vi "HEWH Update Station Message Heating.vi"(6 "Test Complete":bool, 8 "error in (no error)":errorcluster, 10 "Station Label":string, 11 "Display Data (RLT)":T1 {"Current Display" format="%.2f"; "Cycle Count Display" format="%04d"}) -> (0 "error out":errorcluster)   [LabVIEW 2016]
uses:
  Utility/Save File/Public/Type Definitions/Save File Appliance Display.ctl
  Utility/Save File/Public/Type Definitions/Save File Unit Type.ctl
  Utility/Type Definitions/UTILITY Notifier.ctl
  Utility/Custom Pallet Controls/Custom Pallet String.ctl
  Utility/Save File/Global/Save File Globals HCC.vi
  Utility/Save File/Save File.lvlib
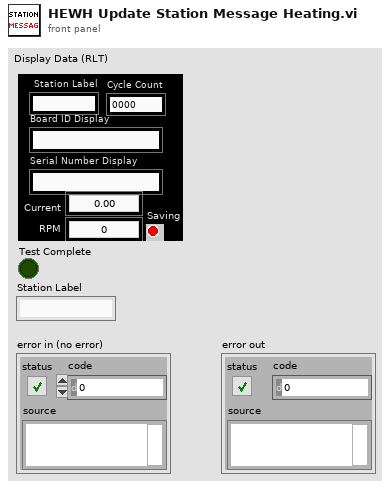
[diagram p1: front panel]
types:
  T1 = typedef "Save File Appliance Display.ctl" = cluster{"Status Color":u32, "Serial Number Display":string, "Cycle Count Display":i32, "Station Label Display":string, "Current Run Start Time Display":dbl, "Board ID Display":string, "RPM Display":u32, "Current Display":dbl, "Current Path Display":path, "Saving Display":bool, "Unit Type Display":T2, "Total Time On Display":dbl, "UI Button":bool}
  T2 = typedef "Save File.lvlib/Save File Unit Type.ctl" = enum32{"", "Viper", "Hawk", "2015"}
  T3 = typedef "UTILITY Notifier.ctl" = enum16{"Set", "Read", "Release Ref"}
  T4 = typedef "Custom Pallet String.ctl" = string
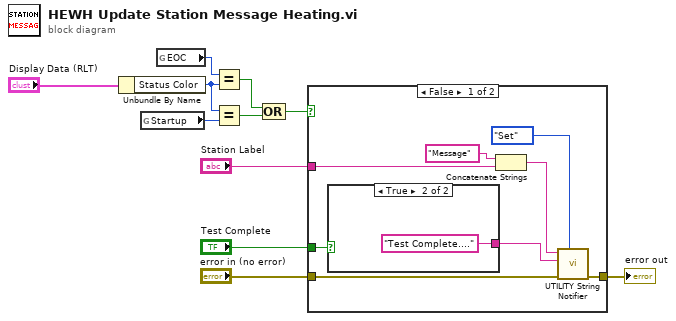
[diagram p0: block diagram]
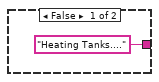
[diagram p2: hidden frame]
diagram:
  n1 = Unbundle By Name("Display Data (RLT)") -> ("Status Color"=w4:u32)
  n2 = global read "Save File Globals HCC.vi" "Startup"() -> (w6:u32)
  n3 = global read "Save File Globals HCC.vi" "EOC"() -> (w3:u32)
  n4 = Equal?(x=w3, y=w4) -> (x = y?=w7:bool)
  n5 = Equal?(x=w4, y=w6) -> (x = y?=w5:bool)
  n6 = Compound Arithmetic op=OR(w7, w5) -> (w2:bool)
  n7 = case shown="False" w2 {
    tunnel: "error in (no error)" -> [w18 w22]
    tunnel: [w17 w22] -> w9
    tunnel: "Station Label" -> [w14 _]
    tunnel: "Test Complete" -> [w12 _]
    frame False {
      n8 = case shown="True" w12 {
        tunnel: [T4 "Heating Tanks...." ("Message") T4 "Test Complete...." ("Message")] -> w16
        frame False {
        }
        frame True {
        }
      }
      n9 = Concatenate Strings("Message" ("name (unnamed)"), w14) -> (w13:string)
      n10 = call "UTILITY String Notifier.vi"("Status"=UTILITY_Notifier."Set", "error in (no error)"=w18, "Set Status"=w16, "name (unnamed)"=w13) -> ("error out"=w17:errorcluster)  [unwired: 6 in, 1 out]
    }
    frame True {
    }
  }
  "error out" <- w9
